vi "NISE.Get Physical Channel Property (1D DBL).vi"(0 "SLSC Interface in":refnum<class "SLSC Interface.lvclass">, 5 "physical channels":refnum<k21>, 7 "property":refnum<k21>, 11 "error in (no error)":errorcluster) -> (4 "SLSC Interface out":refnum<class "SLSC Interface.lvclass">, 10 "property value":dbl[](array[numeric]), 15 "error out":errorcluster)   [LabVIEW 2016, in "SLSC Interface.lvclass"]
uses:
  SLSC Interface.lvclass
  NISE.Property Type.ctl
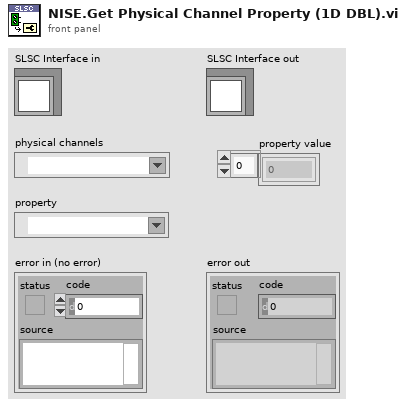
[diagram p1: front panel]
types:
  T1 = typedef "SLSC Interface.lvclass/NISE.Property Type.ctl" = enum16{"Bool", "DBL", "I32", "I64", "String", "U32", "U64", "1D Bool", "1D DBL", "1D I32", "1D I64", "1D String", "1D U32", "1D U64"}
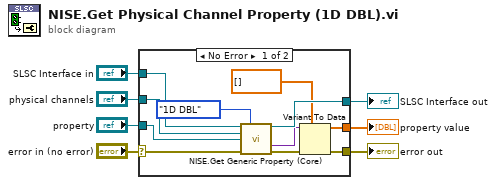
[diagram p0: block diagram]
diagram:
  n1 = case shown="No Error" "error in (no error)" {
    selector: "error in (no error)" -> [w12 w20]
    tunnel: [w11 w20] -> w6
    tunnel: [w17 w19] -> w4
    tunnel: "SLSC Interface in" -> [w18 w19]
    tunnel: "physical channels" -> [w9 _]
    tunnel: "property" -> [w10 _]
    tunnel: [w8 _] -> w1
    frame No Error {
      n2 = call "NISE.Get Generic Property (Core).vi"("SLSC Interface in"=w18, "property type"=NISE.Property_Type."1D DBL", "resources"=w9, "property"=w10, "error in (no error)"=w12) -> ("SLSC Interface out"=w17:refnum<class "SLSC Interface.lvclass">, "property value"=w15:variant, "error out"=w13:errorcluster)  [unwired: 8 in]
      n3 = Variant To Data(error in=w13, type=dbl[] [], Variant=w15) -> (data=w8:dbl[], error out=w11:errorcluster)
    }
    frame Error {
    }
  }
  "error out" <- w6
  "SLSC Interface out" <- w4
  "property value" <- w1
